vi "Spawn.vi"(6 "Round":i32, 7 "Runner in":refnum<class "Formation.lvclass">, 9 "Direction":T1, 10 "Parent Idx":i32, 11 "Board":refnum<data-value>) -> (3 "Replicated":refnum<class "Formation.lvclass">)   [LabVIEW 2015, in "Formation.lvclass"]
uses:
  Formation.lvclass
  Board Cluster.ctl
  Type Defs/Direction Enum.ctl
  DVR Data Cluster.ctl
  Formation.lvclass/Formation.ctl
  Type Defs/SB Type Defs.lvlib
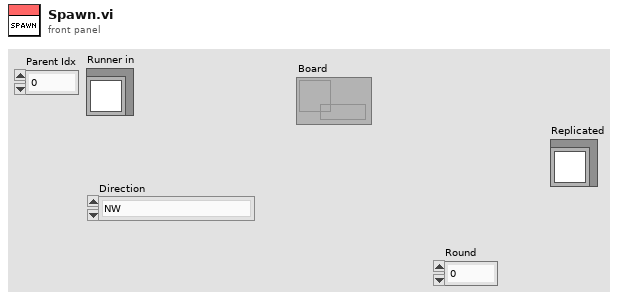
[diagram p1: front panel]
types:
  T1 = typedef "SB Type Defs.lvlib/Direction Enum.ctl" = enum16{"NW", "N", "NE", "E", "SE", "S", "SW", "W"}
  T2 = typedef "Formation.lvclass/DVR Data Cluster.ctl" = cluster{"Moved[Id]":i64, "UnitRound":i32, "Direction":T1, "FormIdx":i32, "LastSpawn":i32, "Spawning?":bool}
  T3 = typedef "Formation.lvclass/Board Cluster.ctl" = cluster{"Board S":i32, "Pos[Idx]":cluster{"X":i32, "Y":i32}[], "Round[Idx]":i32[]}
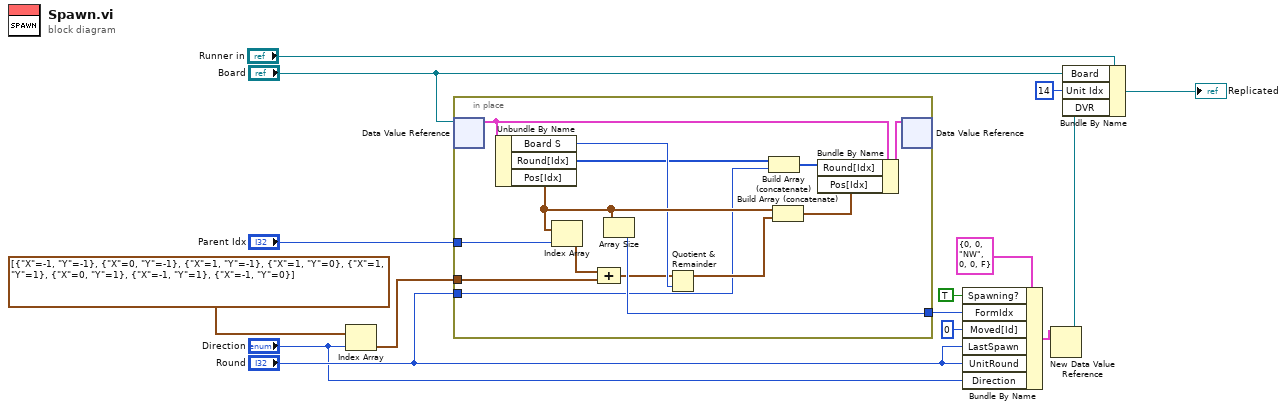
[diagram p0: block diagram]
diagram:
  n1 = Index Array(array=cluster{"X":i32, "Y":i32}[] [{"X"=-1, "Y"=-1}, {"X"=0, "Y"=-1}, {"X"=1, "Y"=-1}, {"X"=1, "Y"=0}, {"X"=1, "Y"=1}, {"X"=0, "Y"=1}, {"X"=-1, "Y"=1}, {"X"=-1, "Y"=0}], index="Direction") -> (element=w2:cluster{"X":i32, "Y":i32})
  n2 = in-place {
    in-place-border: "Parent Idx" -> [w29]
    in-place-border: "Round" -> [w16]
    in-place-border: [w25] -> w4
    in-place-border: w2 -> [w21]
    n3 = in-place-dvr #1("Board") -> (w28:T3)  [unwired: 1 out]
    n4 = Unbundle By Name(w28) -> ("Board S"=w23:i32, "Round[Idx]"=w18:i32[], "Pos[Idx]"=w26:cluster{"X":i32, "Y":i32}[])
    n5 = Index Array(array=w26, index=w29) -> (element=w22:cluster{"X":i32, "Y":i32})
    n6 = Compound Arithmetic op=ADD(w22, w21) -> (w20:cluster{"X":i32, "Y":i32})
    n7 = Array Size(array=w26) -> (size(s)=w25:i32)
    n8 = Quotient & Remainder(x=w20, y=w23) -> (x-y*floor(x/y)=w19:cluster{"X":i32, "Y":i32})  [unwired: 1 out]
    n9 = Build Array (concatenate)(w18, w16) -> (w17:i32[])
    n10 = Build Array (concatenate)(w26, w19) -> (w24:cluster{"X":i32, "Y":i32}[])
    n11 = Bundle By Name(cluster=w28, "Round[Idx]"=w17, "Pos[Idx]"=w24) -> (w27:T3)
    n12 = in-place-dvr #1(w27) -> ()  [unwired: 2 out]
  }
  n13 = Bundle By Name(cluster=T2 {"Moved[Id]"=0, "UnitRound"=0, "Direction"=enum."NW", "FormIdx"=0, "LastSpawn"=0, "Spawning?"=FALSE} ("Cluster"), "Spawning?"=TRUE, "FormIdx"=w4, "Moved[Id]"=i64 0, "LastSpawn"="Round", "UnitRound"="Round", "Direction"="Direction") -> (w14:T2)
  n14 = New Data Value Reference(data value=w14) -> (data value reference=w10:refnum<data-value>)  [unwired: 1 in, 1 out]
  n15 = Bundle By Name(cluster="Runner in", "Board"="Board", "Unit Idx"=u16 14, "DVR"=w10) -> (→"Replicated":refnum<class "Formation.lvclass">)
